vi "Unpack (if allowable).vi"(11 "CancelableObserver in":refnum<class "CancelableObserver.lvclass">) -> (2 "Array out":refnum<class "Send.lvclass">[](array[class]))   [LabVIEW 2011, in "Messenging.lvlib" / "CancelableObserver.lvclass"]
uses:
  CancelableObserver.lvclass
  Send/Send.lvclass
  CancelableObserver.lvclass/CancelableObserver.ctl
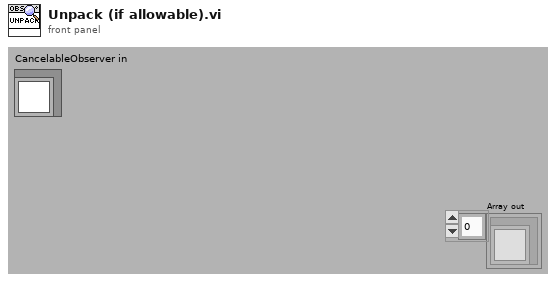
[diagram p1: front panel]
types:
  T1 = typedef "Semaphore RefNum" = refnum<k1>
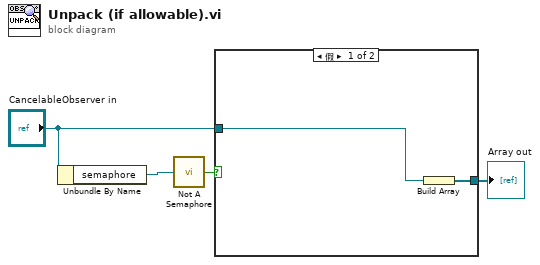
[diagram p0: block diagram]
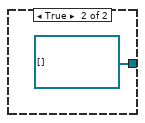
[diagram p2: hidden frame]
diagram:
  n1 = Unbundle By Name("CancelableObserver in") -> ("semaphore"=w4:T1)
  n2 = call <vilib>:"Not A Semaphore.vi"("semaphore"=w4) -> ("not a semaphore"=w3:bool)
  n3 = case shown="假" w3 {
    tunnel: [w6 refnum<class "Send.lvclass">[] [] ("Array out")] -> w2
    tunnel: "CancelableObserver in" -> [w5 _]
    frame False {
      n4 = Build Array(w5) -> (w6:refnum<class "CancelableObserver.lvclass">[])
    }
    frame True {
    }
  }
  "Array out" <- w2
